vi "UploadtoArduino.vi"(10 "serial port":string) -> (2 "standard error":string, 3 "standard output":string)   [LabVIEW 2020]
panel:
  out "resulting string":string
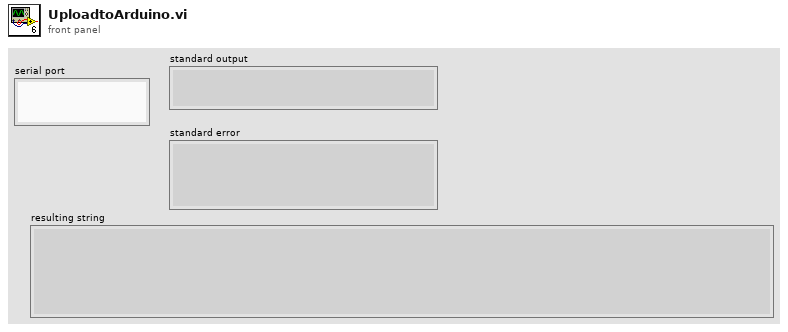
[diagram p1: front panel]
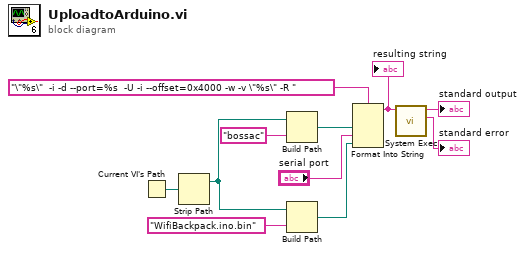
[diagram p0: block diagram]
diagram:
  n1 = Current VI's Path() -> (path=w2:path)
  n2 = Strip Path(path=w2) -> (stripped path=w1:path)  [unwired: 1 out]
  n3 = Build Path(base path=w1, name or relative path="bossac" ("Sketch.ino")) -> (appended path=w3:path)
  n4 = Build Path(base path=w1, name or relative path="WifiBackpack.ino.bin" ("Sketch.ino")) -> (appended path=w7:path)
  n5 = Format Into String(format string="\"%s\"  -i -d --port=%s  -U -i --offset=0x4000 -w -v \"%s\" -R ", w3, "serial port", w7) -> (resulting string=w5:string)  [unwired: 2 in, 1 out]
  "resulting string" <- w5
  n6 = call <vilib>:"System Exec.vi"("command line"=w5) -> ("standard error"=→"standard error":string, "standard output"=→"standard output":string)  [unwired: 7 in, 2 out]
